vi "PM100D_GetSystemInfo.vi"(0 "VISA in":refnum<visa-resource-name>, 1 "error in":errorcluster) -> (2 "VISA out":refnum<visa-resource-name>, 3 "Instrument":string, 4 "SN":string, 5 "error out":errorcluster)   [LabVIEW 2014]
doc: "Get device name and serial number"
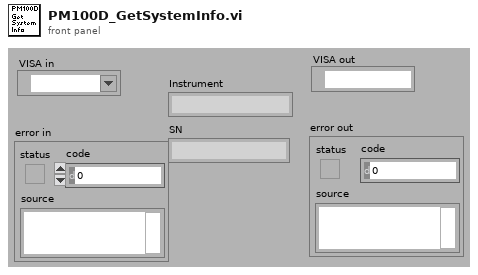
[diagram p1: front panel]
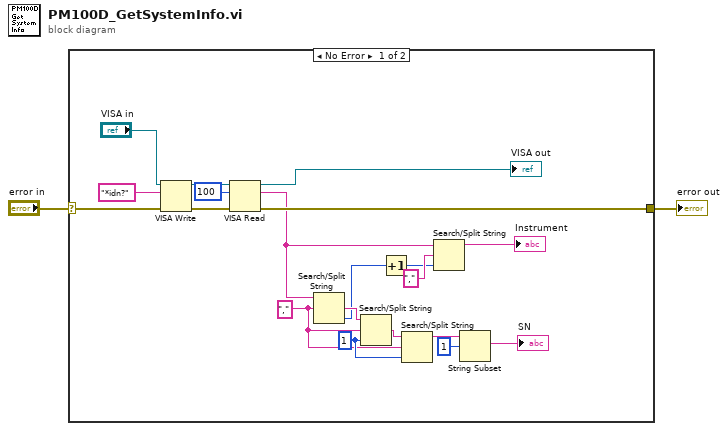
[diagram p0: block diagram]
diagram:
  n1 = case shown="No Error" "error in" {
    selector: "error in" -> [w3 w23]
    tunnel: [w13 w23] -> w2
    frame No Error {
      w19 = 1 ("offset (0)")
      w18 = "," ("search string/char (-)")
      n2 = VISA Write(VISA resource name="VISA in", write buffer="*idn?", error in (no error)=w3) -> (VISA resource name out=w11:refnum<visa-resource-name>, error out=w14:errorcluster)  [unwired: 1 out]
      n3 = VISA Read(VISA resource name=w11, byte count=u32 100, error in (no error)=w14) -> (VISA resource name out=→"VISA out":refnum<visa-resource-name>, read buffer=w8:string, error out=w13:errorcluster)  [unwired: 1 out]
      n4 = Search/Split String(string=w8, search string/char (-)=w18) -> (match + rest of string=w16:string, offset of match=w4:i32)  [unwired: 2 out]
      n5 = Search/Split String(string=w16, search string/char (-)=w18, offset (0)=w19) -> (match + rest of string=w17:string)  [unwired: 2 out]
      n6 = Increment(x=w4) -> (x+1=w6:i32)
      n7 = Search/Split String(string=w17, search string/char (-)=w18, offset (0)=w19) -> (substring before match=w20:string)  [unwired: 2 out]
      n8 = Search/Split String(string=w8, search string/char (-)=",", offset (0)=w6) -> (substring before match=→"Instrument":string)  [unwired: 2 out]
      n9 = String Subset(string=w20, offset (0)=1) -> (substring=→"SN":string)  [unwired: 1 out]
    }
    frame Error {
    }
  }
  "error out" <- w2
